vi "insert.vi"(7 "tree (dvr) in":refnum<data-value>, 8 "error in (no error)":errorcluster, 10 "Data":T2, 11 "Key":T1) -> (0 "error out":errorcluster, 2 "Updated?":bool, 3 "Inserted?":bool)   [LabVIEW 2015, in "binary_tree.lvlib"]
uses:
  binary_tree.lvlib
  _controls/node_data.ctl
  _controls/node_key.ctl
  _controls/tree.ctl
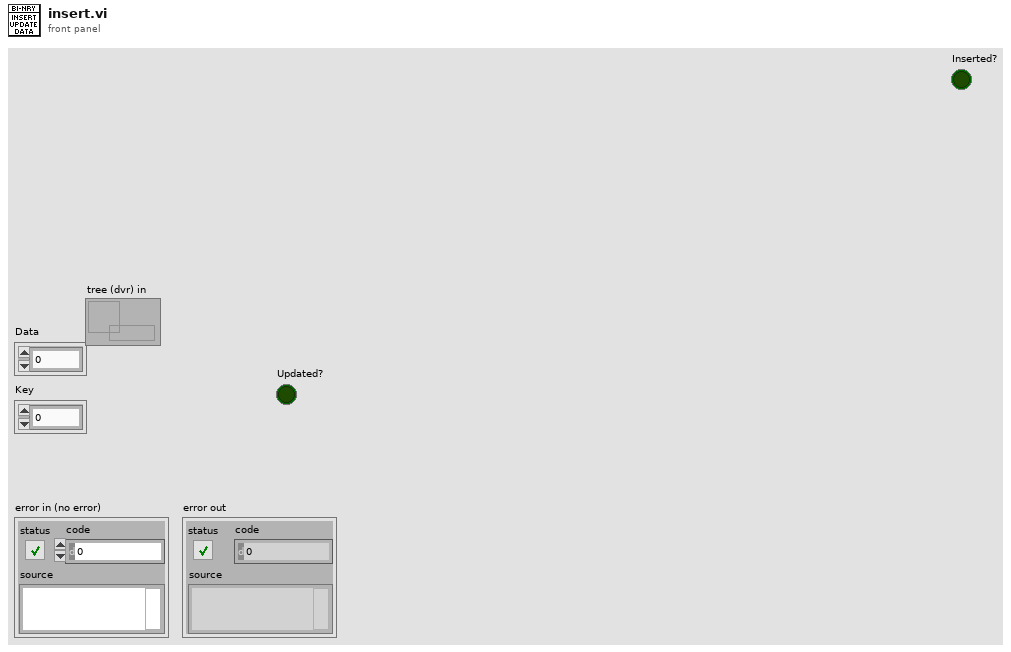
[diagram p1: front panel]
types:
  T1 = typedef "binary_tree.lvlib/node_key.ctl" = cluster{dbl}
  T2 = typedef "binary_tree.lvlib/node_data.ctl" = cluster{dbl}
  T3 = typedef "binary_tree.lvlib/tree.ctl" = cluster{"key":T1, "data":T2, "node_dvr (left)":variant, "node_dvr (right)":variant}
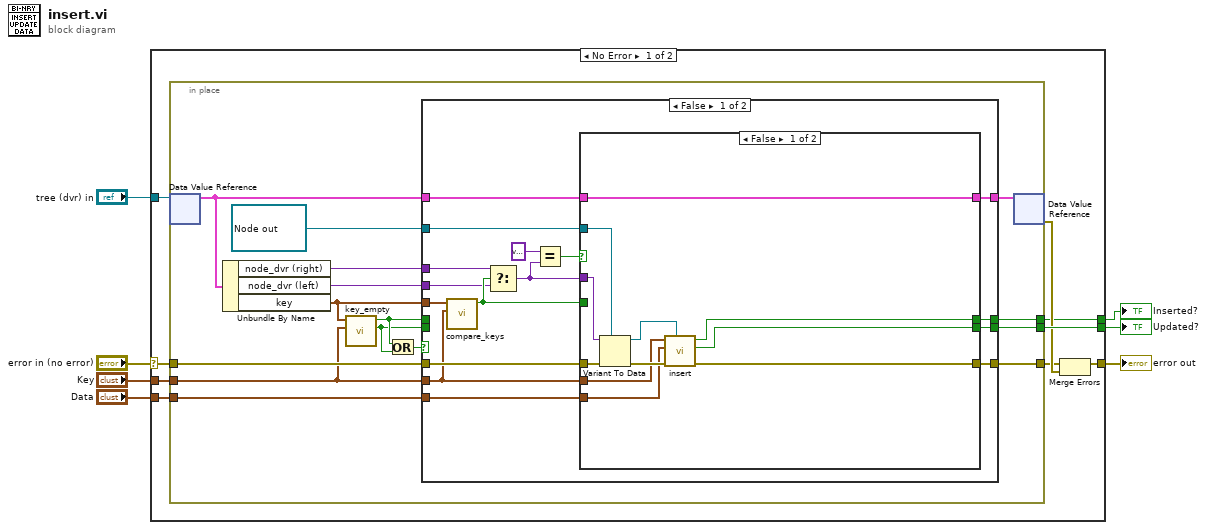
[diagram p0: block diagram]
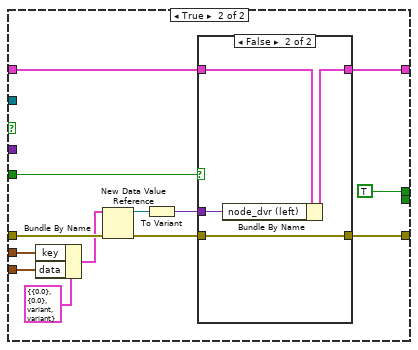
[diagram p2: hidden frame]
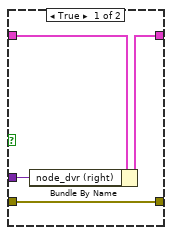
[diagram p3: hidden frame]
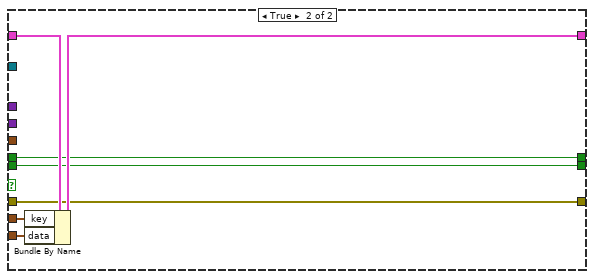
[diagram p4: hidden frame]
diagram:
  n1 = case shown="No Error" "error in (no error)" {
    selector: "error in (no error)" -> [w11 w87]
    tunnel: [w12 w87] -> w7
    tunnel: [w16 _] -> w2
    tunnel: "tree (dvr) in" -> [w15 _]
    tunnel: "Data" -> [w9 _]
    tunnel: "Key" -> [w10 _]
    tunnel: [w8 _] -> w1
    frame No Error {
      n2 = in-place {
        in-place-border: w11 -> [w31]
        in-place-border: [w30] -> w13
        in-place-border: [w29] -> w16
        in-place-border: w10 -> [w19]
        in-place-border: w9 -> [w27]
        in-place-border: [w24] -> w8
        n3 = in-place-dvr #1(w15) -> (w26:T3)  [unwired: 1 out]
        n4 = Unbundle By Name(w26) -> ("node_dvr (right)"=w23:variant, "node_dvr (left)"=w22:variant, "key"=w21:T1)
        n5 = call "key_empty.vi"("Key (search)"=w19, "Key (node)"=w21) -> ("Equal?"=w17:bool, "Empty?"=w18:bool)  [unwired: 8 in]
        n6 = Or(x=w18, y=w17) -> (x .or. y?=w20:bool)
        n7 = case shown="False" w20 {
          tunnel: w21 -> [w47 _]
          tunnel: w31 -> [w46 w81]
          tunnel: [w44 w81] -> w30
          tunnel: [w43 w82] -> w29
          tunnel: refnum<data-value> refnum ("tree (dvr)") -> [w42 _]
          tunnel: w27 -> [w41 w84]
          tunnel: w26 -> [w40 w86]
          tunnel: [w39 w85] -> w25
          tunnel: w19 -> [w38 w80]
          tunnel: [w36 w83] -> w24
          tunnel: w23 -> [w35 _]
          tunnel: w22 -> [w34 _]
          tunnel: w18 -> [_ w83]
          tunnel: w17 -> [_ w82]
          frame False {
            n8 = call "compare_keys.vi"("key (search)"=w38, "key (node)"=w47) -> ("left_right"=w37:bool)  [unwired: 8 in, 1 out]
            n9 = Select(t=w35, s=w37, f=w34) -> (s? t:f=w45:variant)
            n10 = Equal?(x=variant ("Left"), y=w45) -> (x = y?=w33:bool)
            n11 = case shown="False" w33 {
              tunnel: w46 -> [w58 w71]
              tunnel: w45 -> [w57 _]
              tunnel: [w55 w60] -> w44
              tunnel: [w48 _] -> w43
              tunnel: w42 -> [w53 _]
              tunnel: w38 -> [w52 w66]
              tunnel: w40 -> [w51 w68]
              tunnel: [w51 w62] -> w39
              tunnel: w37 -> [_ w64]
              tunnel: w41 -> [w50 w67]
              tunnel: [w49 TRUE] -> w36
              frame False {
                n12 = Variant To Data(error in=w58, type=w53, Variant=w57) -> (data=w54:refnum<data-value>, error out=w56:errorcluster)
                n13 = call "insert.vi"("tree (dvr) in"=w54, "error in (no error)"=w56, "Data"=w50, "Key"=w52) -> ("error out"=w55:errorcluster, "Updated?"=w48:bool, "Inserted?"=w49:bool)  [unwired: 5 in]
              }
              frame True {
                n14 = Bundle By Name(cluster=T3 {"key"={0.0}, "data"={0.0}, "node_dvr (left)"=variant, "node_dvr (right)"=variant} ("data value"), "key"=w66, "data"=w67) -> (w70:T3)
                n15 = New Data Value Reference(data value=w70, error in=w71) -> (data value reference=w65:refnum<data-value>, error out=w61:errorcluster)
                n16 = To Variant(anything=w65) -> (Variant=w63:variant)
                n17 = case shown="False" w64 {
                  tunnel: w68 -> [w75 w79]
                  tunnel: w63 -> [w74 w78]
                  tunnel: [w73 w77] -> w62
                  tunnel: w61 -> [w72 w76]
                  tunnel: [w72 w76] -> w60
                  frame True {
                    n18 = Bundle By Name(cluster=w75, "node_dvr (right)"=w74) -> (w73:T3)
                  }
                  frame False {
                    n19 = Bundle By Name(cluster=w79, "node_dvr (left)"=w78) -> (w77:T3)
                  }
                }
              }
            }
          }
          frame True {
            n20 = Bundle By Name(cluster=w86, "key"=w80, "data"=w84) -> (w85:T3)
          }
        }
        n21 = in-place-dvr #1(w25) -> (w14:errorcluster)  [unwired: 1 out]
      }
      n22 = Merge Errors(w13, w14) -> (w12:errorcluster)
    }
    frame Error {
    }
  }
  "error out" <- w7
  "Updated?" <- w2
  "Inserted?" <- w1
